vi "Intake Controller.vi"(8 "error in":errorcluster) -> ()   [LabVIEW 2019]
doc: "This VI executes continuously carrying out the current operation and responding to updates or new operations. It will often contain the timing or control code that is difficult to place directly in TeleOp. This VI generally opens all sensors and motors and isolates the rest of the robot code from knowing how the operations are carried out."
uses:
  <vilib>/Rock Robotics/WPI/Framework/Completion Status.ctl
  Intake Setpoints.ctl
  Intake Operations.ctl
  <vilib>/Rock Robotics/WPI/ThirdParty/REV Robotics/SPARK MAX/Typedef/Spark MAX Control Type.ctl
  <vilib>/Rock Robotics/WPI/ThirdParty/Phoenix-LabVIEW/Motor Controller/Controls/CTRE_Phoenix_MotorControl_ControlMode.ctl
  <vilib>/Rock Robotics/Network Tables/NT Write Boolean.vi
panel:
  in  "Interactive Values":T1
  out "Current\nCmd":string
  in  "Buttons":cluster{"Execute Cmd":bool, "Abort Cmd":bool}
  out "Command Timing":cluster{"Start Time (ms)":u32, "Iterations":i32}
  out "Status":T3
  # "Tip: It may be helpful to observe inputs and sensor values.\nYou may also want to display tuning or debugging controls."
  # "Interactive Command: You may fill in the settings for a command\nand schedule it with the Execute button. You can observe and abort\nany command while fine tuning the code for the controller."
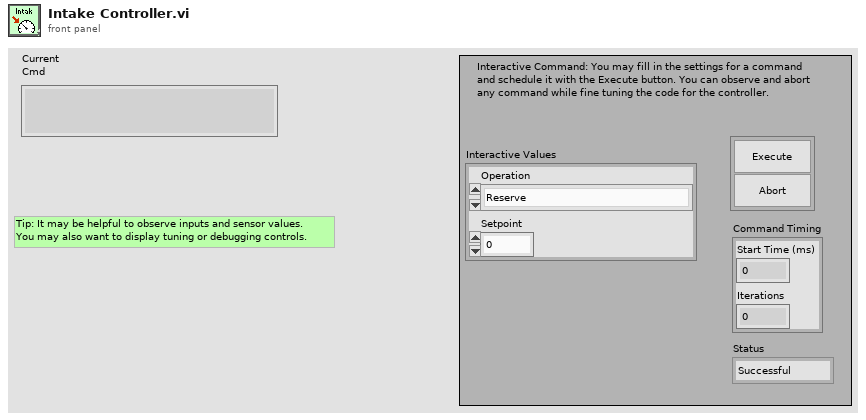
[diagram p1: front panel]
types:
  T1 = typedef "Intake Setpoints.ctl" = cluster{"Operation":T2, "Setpoint":dbl}
  T2 = typedef "Intake Operations.ctl" = enum16{"Reserve", "Read Current", "Immediate"}
  T3 = typedef "Completion Status.ctl" = enum16{"Successful", "Aborted", "Incomplete"}
  T4 = typedef "WPI_MotorControlDeviceRef.ctl" = cluster{"DeviceStatus":errorcluster, "Type":T5, "PWM":cluster{"PWM Channel":T6, "DeadBand":T7}, "CAN":cluster{"Device Number":u8, "SetOutput VI Ref":variant, "GetOutput VI Ref":variant, "Enable VI Ref":variant, "Disable VI Ref":variant, "Data":variant}, "Invert":bool, "DIO PWM":cluster{"PWM \"Enable\" Channel":T6, "DIOChannel":T8, "PWM Rate":dbl}}
  T5 = typedef "WPI_MotorControlType.ctl" = enum16{"PWM", "CAN", "DIO PWM"}
  T6 = typedef "FPGA_DIOPWMChannel.ctl" = enum8{"PWM 0", "PWM 1", "PWM 2", "PWM 3", "PWM 4", "PWM 5", "PWM 6", "PWM 7", "PWM 8", "PWM 9", "PWM MXP 0", "PWM MXP 1", "PWM MXP 2", "PWM MXP 3", "PWM MXP 4", "PWM MXP 5", "PWM MXP 6", "PWM MXP 7", "PWM MXP 8", "PWM MXP 9", "Invalid"}
  T7 = typedef "WPI_PWMDeadband.ctl" = cluster{"Name":string, "maxPositivePwm":i32, "minPositivePwm":i32, "centerPwm":i32, "maxNegativePwm":i32, "minNegativePwm":i32, "angularRange":u16}
  T8 = typedef "FPGA_DIOChannel.ctl" = enum8{"DIO 0", "DIO 1", "DIO 2", "DIO 3", "DIO 4", "DIO 5", "DIO 6", "DIO 7", "DIO 8", "DIO 9", "DIO MXP 0", "DIO MXP 1", "DIO MXP 2", "DIO MXP 3", "DIO MXP 4", "DIO MXP 5", "DIO MXP 6", "DIO MXP 7", "DIO MXP 8", "DIO MXP 9", "DIO MXP 10", "DIO MXP 11", "DIO MXP 12", "DIO MXP 13", "DIO MXP 14", "DIO MXP 15", "SPI Port CS1", "SPI Port CS2", "SPI Port CS3", "SPI Port MISO", "SPI Port MOSI", "Invalid"}
  T9 = typedef "Command Status Info.ctl" = cluster{"Name":string, "Status":T3, "notifier out":T10}
  T10 = typedef "Completion Notifier.ctl" = refnum<notifier>
  T11 = cluster{"Current Command":T1, "Command Timing":cluster{"Start Time (ms)":u32, "Iterations":i32}, "Command Arguments":cluster{"Command Info":T9, "Description":string, "Default Command":T1, "queue out":refnum<queue>, "Subsystem Name":string}}
  T12 = typedef "Spark MAX Control Type.ctl" = enum16{"Percent VBus", "Voltage", "Velocity", "Position", "Smart Motion", "Current", "Smart Velocity"}
  T13 = typedef "CTRE_Phoenix_MotorControl_ControlMode.ctl" = u16
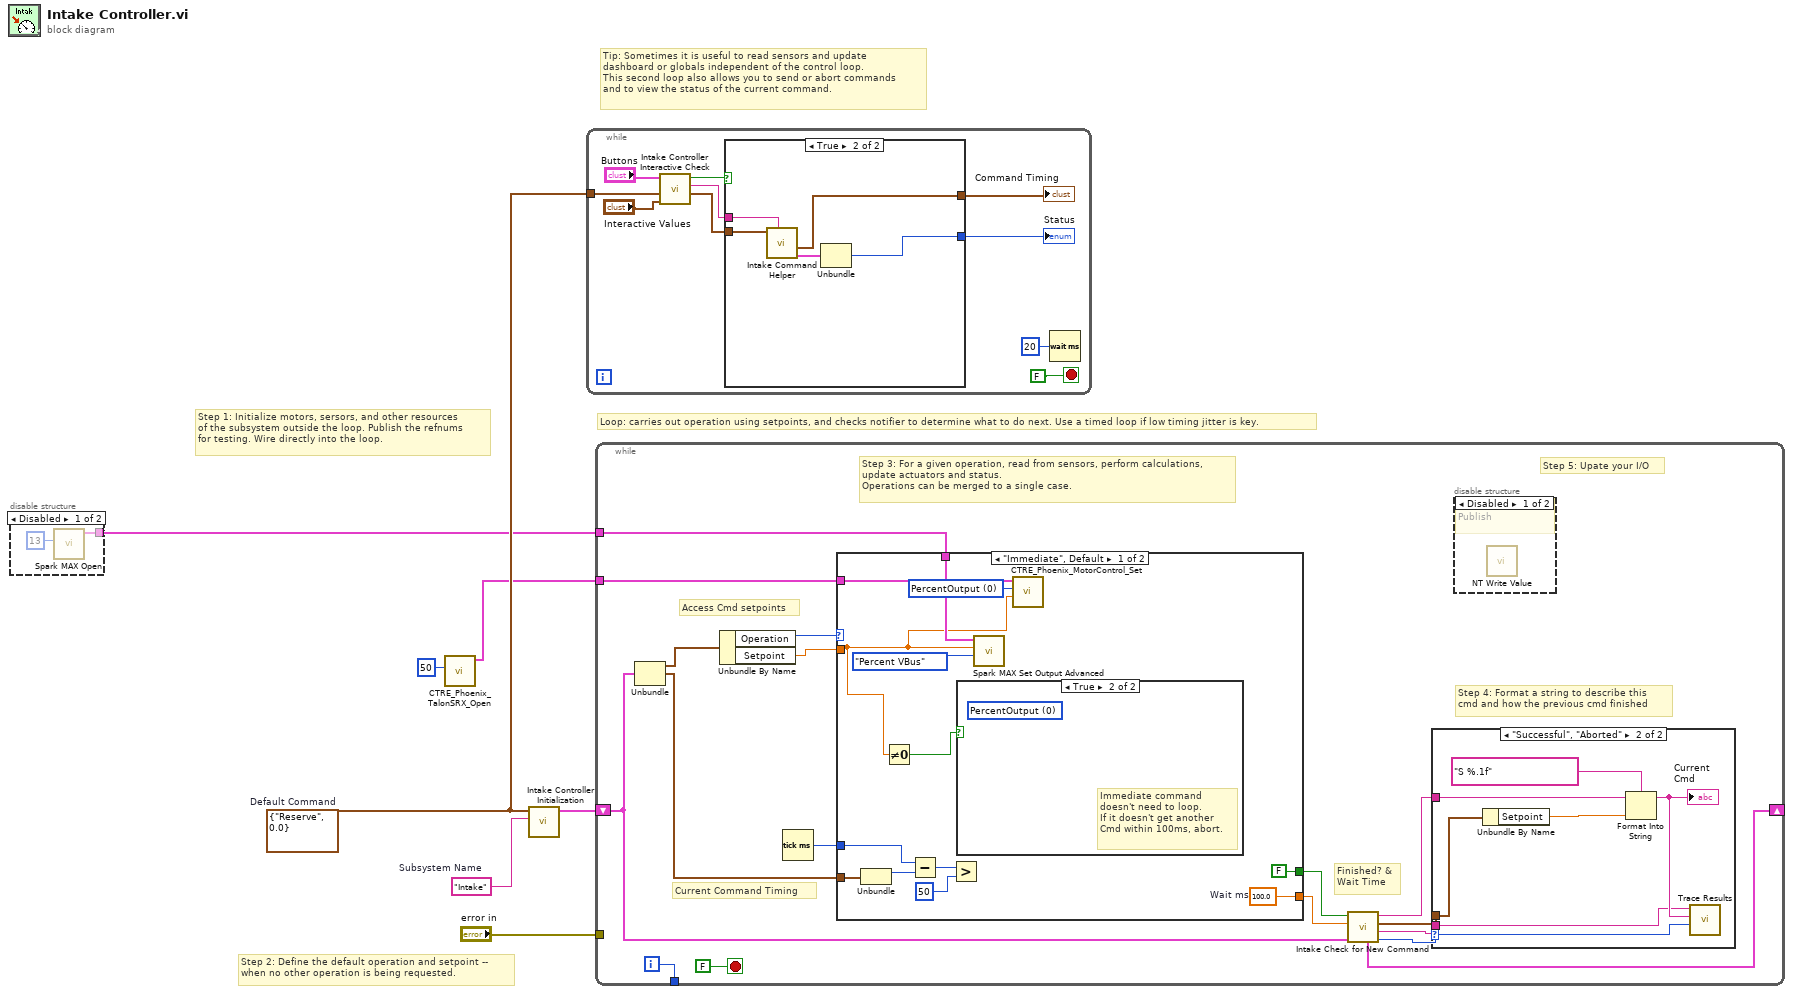
[diagram p0: block diagram]
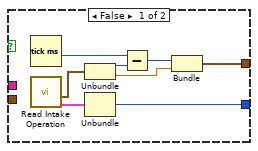
[diagram p3: hidden frame]
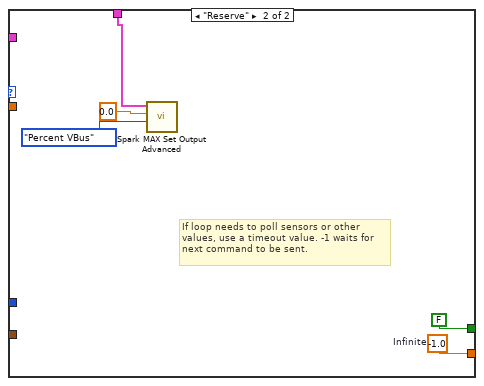
[diagram p7: hidden frame]
diagram:
  w4 = T1 {"Operation"=enum."Reserve", "Setpoint"=0.0}  # Default Command
  w5 = "Intake"  # Subsystem Name
  # "Tip: Sometimes it is useful to read sensors and update\ndashboard or globals independent of the control loop.\nThis second loop also allows you to send or abort commands\nand to view the status of the current command."
  # "Step 2: Define the default operation and setpoint --\nwhen no other operation is being requested."
  # "Step 1: Initialize motors, sersors, and other resources\nof the subsystem outside the loop. Publish the refnums\nfor testing. Wire directly into the loop."
  # "Loop: carries out operation using setpoints, and checks notifier to determine what to do next. Use a timed loop if low timing jitter is key."
  n1 = disable-structure shown="Disabled" {
    disable-tunnel: [w9 _] -> w3
    frame Disabled {
      n2 = call <vilib>:"Spark MAX Open.vi"("Device Number"=u8 13) -> ("MotorControlDeviceRef"=w9:T4)  [unwired: 9 in, 1 out]
    }
    frame Enabled {
    }
  }
  n3 = call <vilib>:"CTRE_Phoenix_TalonSRX_Open.vi"("Device Number"=u8 50) -> ("CAN Talon SRX Ref"=w1:T4)  [unwired: 9 in, 1 out]
  n4 = call "Intake Controller Initialization.vi"("Subsystem Name"=w5, "Default Command"=w4) -> ("Current Command"=w6:T11)  [unwired: 9 in]
  n5 = while {
    tunnel: w4 -> [w16]
    stop <- FALSE stop-if-true
    n6 = call "Intake Controller Interactive Check.vi"("Interactive Command in"="Interactive Values", "Default Command"=w16, "Buttons"="Buttons") -> ("Interactive Command out"=w13:T1, "Trace String"=w14:string, "Schedule"=w15:bool)  [unwired: 6 in]
    n7 = case shown="True" w15 {
      tunnel: [w27 w32] -> w12
      tunnel: w13 -> [_ w30]
      tunnel: [w23 w28] -> w11
      tunnel: w14 -> [_ w31]
      frame False {
        n8 = Tick Count (ms)() -> (millisecond timer value=w22:u32)
        n9 = call "Read Intake Operation.vi"() -> ("Command Info"=w20:T9, "SubSystem Data"=w21:T1)  [unwired: 9 in, 1 out]
        n10 = Unbundle(w21) -> ("Operation"=w26:T2, "Setpoint"=w24:dbl)
        n11 = Unbundle(w20) -> ("Status"=w27:T3)  [unwired: 2 out]
        n12 = Subtract(x=w22, y=w26) -> (x-y=w25:u32)
        n13 = Bundle(w25, "Setpoint"=w24) -> (w23:cluster{u32, "Setpoint":dbl})  [unwired: 1 in]
      }
      frame True {
        n14 = call "Intake Command Helper.vi"("Description"=w31, "SubSystem Data"=w30) -> ("Command Info Out"=w29:T9, "Command Timing"=w28:cluster{"Start Time (ms)":u32, "Iterations":i32})  [unwired: 7 in, 1 out]
        n15 = Unbundle(w29) -> ("Status"=w32:T3)  [unwired: 2 out]
      }
    }
    "Status" <- w12
    "Command Timing" <- w11
    n16 = Wait (ms)(milliseconds to wait=u32 20) -> ()  [unwired: 1 out]
  }
  n17 = while {
    shift-right: [w42] -> _
    shift-left: w6 -> [w35]
    tunnel: [w48] -> _
    tunnel: "error in" -> [_]
    tunnel: w3 -> [w34]
    tunnel: w1 -> [w33]
    i -> [w48]
    stop <- FALSE stop-if-true
    # "Step 5: Upate your I/O"
    # "Step 4: Format a string to describe this\ncmd and how the previous cmd finished"
    # "Current Command Timing"
    # "Access Cmd setpoints"
    # "Finished? &\nWait Time"
    # "Step 3: For a given operation, read from sensors, perform calculations,\nupdate actuators and status.\nOperations can be merged to a single case."
    n18 = Unbundle(w35) -> ("Current Command"=w47:T1, "Command Timing"=w44:cluster{"Start Time (ms)":u32, "Iterations":i32})  [unwired: 1 out]
    n19 = Unbundle By Name(w47) -> ("Operation"=w46:T2, "Setpoint"=w43:dbl)
    n20 = Tick Count (ms)() -> (millisecond timer value=w45:u32)
    n21 = case shown="\"Immediate\", Default" w46 {
      tunnel: [w69 w74] -> w40
      tunnel: [FALSE ("ignore previous (F)") FALSE ("ignore previous (F)")] -> w41
      tunnel: w44 -> [w65 _]
      tunnel: w45 -> [w64 _]
      tunnel: w43 -> [w57 _]
      tunnel: w34 -> [w62 w72]
      tunnel: w33 -> [w59 _]
      frame "Immediate", Default {
        w58 = T13 0 items=["PercentOutput"=0, "Position"=1, "Velocity"=2, "Current"=3, "Follower"=5, "MotionProfile"=6, "MotionMagic"=7, "MotionProfileArc"=10, "Disabled"=15] ("Control Mode")
        w69 = 100.0  # Wait ms
        n22 = Unbundle(w65) -> ("Start Time (ms)"=w68:u32)  [unwired: 1 out]
        n23 = Not Equal To 0?(x=w57) -> (x != 0?=w60:bool)
        n24 = Subtract(x=w64, y=w68) -> (x-y=w67:u32)
        n25 = Greater?(x=w67, y=u8 50 ("Left Motor")) -> ()  [unwired: 1 out]
        n26 = case shown="True" w60 {
          frame False {
          }
          frame True {
            (unwired) T13 0 items=["PercentOutput"=0, "Position"=1, "Velocity"=2, "Current"=3, "Follower"=5, "MotionProfile"=6, "MotionMagic"=7, "MotionProfileArc"=10, "Disabled"=15] ("Control Mode")
            # "Immediate command\ndoesn't need to loop.\nIf it doesn't get another\nCmd within 100ms, abort."
          }
        }
        n27 = call <vilib>:"Spark MAX Set Output Advanced.vi"("Control Mode"=Spark_MAX_Control_Type."Percent VBus", "Setpoint"=w57, "MotorControlDevRef"=w62) -> ()  [unwired: 7 in, 2 out]
        n28 = call <vilib>:"CTRE_Phoenix_MotorControl_Set.vi"("Output"=w57, "Control Mode"=w58, "PhoenixMotorControlDevRef"=w59) -> ()  [unwired: 7 in, 2 out]
      }
      frame "Reserve" {
        w74 = -1.0  # Infinite
        # "If loop needs to poll sensors or other\nvalues, use a timeout value. -1 waits for\nnext command to be sent."
        n29 = call <vilib>:"Spark MAX Set Output Advanced.vi"("Control Mode"=Spark_MAX_Control_Type."Percent VBus", "Setpoint"=0.0, "MotorControlDevRef"=w72) -> ()  [unwired: 7 in, 2 out]
      }
    }
    n30 = call "Intake Check for New Command.vi"("Current Command"=w35, "Wait time (ms)"=w40, "Finished?"=w41) -> ("Completion"=w36:T3, "Subsystem Name"=w37:string, "Current Command"=w38:T1, "Initial Trace String"=w39:string, "NextCommand"=w42:T11)  [unwired: 4 in]
    n31 = case shown="\"Successful\", \"Aborted\"" w36 {
      selector: w36 -> [_ w56]
      tunnel: w39 -> [_ w52]
      tunnel: w38 -> [_ w53]
      tunnel: w37 -> [_ w50]
      frame "Incomplete", Default {
        # "Continuing current command"
      }
      frame "Successful", "Aborted" {
        # "Report and setup for next command"
        n32 = Unbundle By Name(w53) -> ("Setpoint"=w55:dbl)
        n33 = Format Into String(format string="S %.1f", initial string=w52, w55) -> (resulting string=w51:string)  [unwired: 1 in, 1 out]
        "Current\nCmd" <- w51
        n34 = call <vilib>:"Trace Results.vi"("Status of previous command"=w56, "Description"=w51, "Subsystem"=w50) -> ()  [unwired: 9 in]
      }
    }
    n35 = disable-structure shown="Disabled" {
      frame Disabled {
        # "Publish"
        n36 = call-poly <vilib>:"NT Write Value.vi"() -> ()  [unwired: 11 in, 1 out]
      }
      frame Enabled {
      }
    }
  }
